vi "Bounds to Size.vi"(11 "bounds":T2) -> (3 "size":T1)   [LabVIEW 2010, in "NI_SE_Front Panel Layout.lvlib"]
uses:
  NI_SE_Front Panel Layout.lvlib
  <vilib>/Utility/miscctls.llb/LVRectTypeDef.ctl
  <vilib>/Utility/miscctls.llb/LVPointTypeDef.ctl
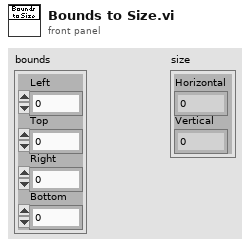
[diagram p1: front panel]
types:
  T1 = typedef "LVPointTypeDef.ctl" = cluster{"Horizontal":i16, "Vertical":i16}
  T2 = typedef "LVRectTypeDef.ctl" = cluster{"Left":i16, "Top":i16, "Right":i16, "Bottom":i16}
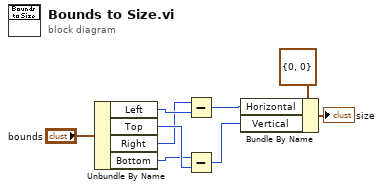
[diagram p0: block diagram]
diagram:
  n1 = Unbundle By Name("bounds") -> ("Left"=w7:i16, "Top"=w9:i16, "Right"=w6:i16, "Bottom"=w8:i16)
  n2 = Subtract(x=w6, y=w7) -> (x-y=w3:i16)
  n3 = Subtract(x=w8, y=w9) -> (x-y=w2:i16)
  n4 = Bundle By Name(cluster=T1 {"Horizontal"=0, "Vertical"=0} ("Point"), "Horizontal"=w3, "Vertical"=w2) -> (→"size":T1)
